vi "RT_AIChar_v3.vi"() -> ()   [LabVIEW 2020]
uses:
  <vilib>/NI/STM/SubVIs/MetaDataElement.ctl
  <vilib>/Platform/TimedLoop/XDataNode/timing_clust.ctl
  <vilib>/Platform/TimedLoop/XDataNode/nitl_modes.ctl
  <vilib>/Platform/TimedLoop/XDataNode/wakeup.ctl
  <vilib>/NI/STM/TCP/Write Meta Data (TCP Ref).vi
  <vilib>/NI/STM/TCP/Get Connection Reference (TCP).vi
  <vilib>/NI/STM/TCP/Write Meta Data (TCP Clst).vi
  <vilib>/FPGAPlugInAG/cRIO-9049/niLvFpga_Open_cRIO-9049.vi
  <vilib>/rvi/interface/common/dynamic/niFpgaDynamicAddResources.vi
  <vilib>/NI/STM/TCP/Write Message (TCP).vi
  <vilib>/Utility/error.llb/Error Cluster From Error Code.vi
  <vilib>/rvi/errors/niLvFpgaAdjustHostInterfaceError.vi
  <vilib>/FPGAPlugInAG/Dynamic/niLvFpga_Close_Dynamic.vi
  <vilib>/rvi/interface/nirviOpenFPGA/nirviOpenFPGA.xnode
  FPGA Bitfiles/levitationcode_FPGATarget_FPGAmainCtrlv4_ym4N2scWarI.lvbitx
  <vilib>/Platform/TimedLoop/XDataNode/XDataNode.xnode
  <vilib>/rvi/interface/nirviReadWriteControl/nirviReadWriteControl.xnode
  <vilib>/rvi/interface/nirviCloseFPGA/nirviCloseFPGA.xnode
  <vilib>/Platform/TimedLoop/XDataNode/XDNodeRunTimeDep.lvlib
  Components_global/Timing/Timing.lvlib
  <vilib>/NI/STM/NI STM.lvlib
  <vilib>/rvi/interface/Simulation/niFpgaSimulationCallBeginRW.vi
  NiFpgaLv.dll
panel:
  in  "Select channel":T1(ring)
  in  "Select HS or LS?":enum16{"HS (NI9222)", "LS (NI9220)"}(ring)
  out "RT Loop Rate":dbl format="%.3p"
  out "# of iterations\n[STM write]":i32
  out "# elements \nFIFO buffer":u32
  out "Finished \nlate counter?":dbl
  in  "stop":bool
  # "- Open PC_SensorChar vi and run that VI as well to start capturing data!"
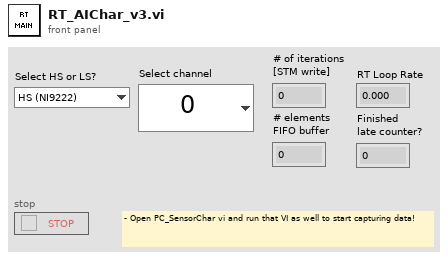
[diagram p1: front panel]
types:
  T1 = enum16{"0", "1", "2", "3", "4", "5", "6", "7", "8", "9", "10", "11", "12", "13", "14", "15"}
  T2 = typedef "NI STM.lvlib/MetaDataElement.ctl" = string
  T3 = typedef "NI STM.lvlib/TCP Connection Info.ctl" = cluster{"connection ID":refnum<k5>, "meta data":T2[]}
  T4 = typedef "XDNodeRunTimeDep.lvlib/timing_clust.ctl" = cluster{"Expected End [f-1]":u64, "Actual End [f-1]":u64, "Finished Late? [f-1]":bool, "Expected End [i-1]":u64, "Actual End [i-1]":u64, "Finished Late? [i-1]":bool, "Expected Start [i]":u64, "Actual Start [i]":u64, "Expected Start [f]":u64, "Actual Start [f]":u64, "Source Name":string, "Structure Name":string, "Period":i64, "Deadline":i64, "Offset":i64, "Start":i64, "Priority":i32, "Timeout":i32, "Mode":T5, "Wakeup Reason":T6, "Error":errorcluster, "Source Type":string, "Secondary Source Type":string, "Global End Time":u64, "Global Start Time":u64, "Frame Duration":u64, "Iteration Duration":u64, "Assigned CPU":i32, "I/O Scan Engine Mode":u32}
  T5 = typedef "XDNodeRunTimeDep.lvlib/nitl_modes.ctl" = enum32{"No Change", "Process missed periods, maintain original phase", "Discard missed periods, maintain original phase", "Process missed periods, ignore original phase", "Discard missed periods, ignore original phase"}
  T6 = typedef "XDNodeRunTimeDep.lvlib/wakeup.ctl" = enum32{"Normal", "Aborted", "Asynchronous wakeup", "Timing source error", "Timed loop error", "Timeout"}
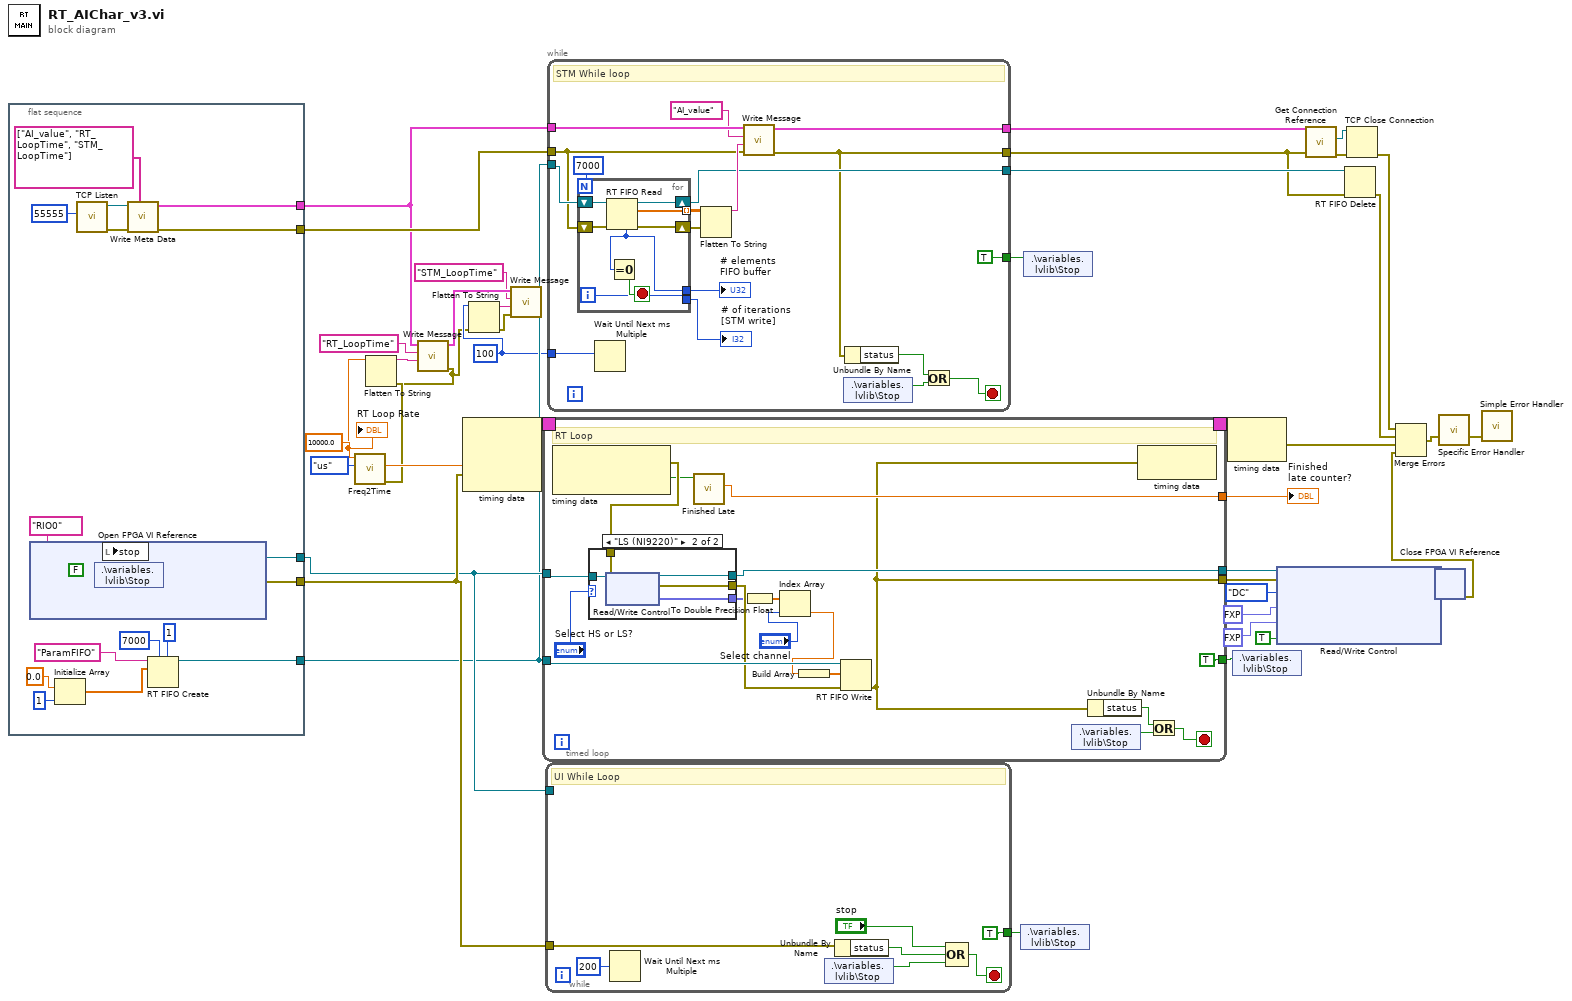
[diagram p0: block diagram]
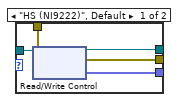
[diagram p2: hidden frame]
diagram:
  w11 = u32 100 ("millisecond multiple")
  n1 = flat-sequence {
    tunnel: [w59] -> w22
    tunnel: [w58] -> w21
    tunnel: [w53] -> w8
    tunnel: [w52] -> w37
    tunnel: [w51] -> w12
    frame #0 {
      w60 = FALSE ("Stop")
      n2 = xnode "Open FPGA VI Reference"("resource name"=tag "RIO0") -> ("FPGA VI Reference Out"=w58:refnum<k20>, "error out"=w61:errorcluster)  [unwired: 1 in]
      n3 = Initialize Array(0.0 ("element"), 1 ("dimension size")) -> (w46:dbl[])
      n4 = call <vilib>:"TCP Listen.vi"("port"=u16 55555) -> ("error out"=w56:errorcluster, "connection ID"=w55:refnum<k5>)  [unwired: 6 in, 3 out]
      n5 = shared-variable ".\\variables.lvlib\\Stop"(w60, error in=w61) -> (error out=w59:errorcluster)
      n6 = local write "stop"(w60) -> ()
      n7 = call-poly <vilib>:"Write Meta Data.vi"("meta data"=T2[] ["AI_value", "RT_LoopTime", "STM_LoopTime"], "error in"=w56, "connection ID"=w55) -> ("error out"=w52:errorcluster, "connection info out"=w53:T3)  [unwired: 7 in]
      n8 = RT FIFO Create(0:"ParamFIFO" ("name (unnamed)"), 1:w46, 4:u32 7000 ("size (10)"), 6:u32 1 ("elements in array (1)")) -> (8:w51:refnum<k33>)  [unwired: 4 in, 2 out]
    }
  }
  n9 = call "Freq2Time.vi"("Int. Time Unit"=enum16{"sec", "us", "ms"}."us", "Sample rate (Hz)"=10000.0 ("Period")) -> ("error out"=w26:errorcluster, "Int.  time [unit]"=w38:dbl, "New Sample rate (Hz)"=w28:dbl)  [unwired: 7 in]
  "RT Loop Rate" <- w28
  n10 = Flatten To String(anything=w28, error in (no error)=w26) -> (data string=w29:string, error out=w10:errorcluster)  [unwired: 2 in, 1 out]
  n11 = call-poly <vilib>:"Write Message.vi"("error in"=w10, "data"=w29, "name"="RT_LoopTime", "connection info in"=w8) -> ("connection info out"=w7:T3)  [unwired: 6 in, 1 out]
  n12 = node-c288(w38, w22) -> (w43:T4)  [unwired: 1 in]
  n13 = Flatten To String(anything=w11, error in (no error)=w10) -> (data string=w5:string, error out=w9:errorcluster)  [unwired: 2 in, 1 out]
  n14 = call-poly <vilib>:"Write Message.vi"("error in"=w9, "data"=w5, "name"="STM_LoopTime", "connection info in"=w7) -> ()  [unwired: 6 in, 2 out]
  n15 = timed-loop {
    tunnel: w21 -> [w79]
    timing: w43 -> [_]
    timing-out: [_] -> w42
    tunnel: [w76] -> w41
    tunnel: w12 -> [w75]
    tunnel: [TRUE ("Stop")] -> w14
    tunnel: [w67] -> w4
    tunnel: [w66] -> w3
    stop <- w73 stop-if-true
    # "RT Loop"
    n16 = node-c288() -> (w78:errorcluster, w77:bool)  [unwired: 1 in]
    n17 = case shown="\"LS (NI9220)\"" "Select HS or LS?" {
      tunnel: w79 -> [w84 w89]
      tunnel: w78 -> [w83 w88]
      tunnel: [w82 w87] -> w65
      tunnel: [w81 w86] -> w67
      tunnel: [w80 w85] -> w69
      frame "HS (NI9222)", Default {
        n18 = xnode "Read/Write Control"("FPGA VI Reference In"=w84, "error in"=w83) -> ("FPGA VI Reference Out"=w81:refnum<k20>, "error out"=w80:errorcluster, "AI_HS"=w82:fxp<+/-,25,5>[])
      }
      frame "LS (NI9220)" {
        n19 = xnode "Read/Write Control"("FPGA VI Reference In"=w89, "error in"=w88) -> ("FPGA VI Reference Out"=w86:refnum<k20>, "error out"=w85:errorcluster, "AI_LS"=w87:fxp<+/-,25,5>[])
      }
    }
    n20 = call "Finished Late.vi"("Finished \nLate?"=w77) -> ("# Finished\nLate counter"=w76:dbl)  [unwired: 8 in, 2 out]
    n21 = To Double Precision Float(number=w65) -> (double precision float=w64:dbl[])
    n22 = Index Array(array=w64, index="Select channel") -> (element=w63:dbl)
    n23 = Build Array(w63) -> (w62:dbl[])
    n24 = RT FIFO Write(0:w75, 1:w62, 3:w69) -> (11:w66:errorcluster)  [unwired: 2 in, 3 out]
    n25 = shared-variable ".\\variables.lvlib\\Stop"() -> (w72:bool)  [unwired: 1 in, 1 out]
    n26 = Unbundle By Name(w66) -> ("status"=w71:bool)
    n27 = node-c288(w66) -> ()  [unwired: 1 out]
    n28 = Or(x=w71, y=w72) -> (x .or. y?=w73:bool)
  }
  "Finished \nlate counter?" <- w41
  n29 = while {
    tunnel: w22 -> [w98]
    tunnel: w21 -> [_]
    tunnel: [TRUE ("Stop")] -> w13
    stop <- w99 stop-if-true
    # "UI While Loop"
    n30 = Wait Until Next ms Multiple(millisecond multiple=u32 200) -> ()  [unwired: 1 out]
    n31 = shared-variable ".\\variables.lvlib\\Stop"() -> (w100:bool)  [unwired: 1 in, 1 out]
    n32 = Unbundle By Name(w98) -> ("status"=w97:bool)
    n33 = Compound Arithmetic op=OR("stop", w97, w100) -> (w99:bool)
  }
  n34 = while {
    tunnel: w8 -> [w120]
    tunnel: w37 -> [w114]
    tunnel: [w118] -> w36
    tunnel: [w104] -> w32
    tunnel: w12 -> [w116]
    tunnel: [w113] -> w33
    tunnel: [TRUE ("Stop")] -> w15
    tunnel: w11 -> [w103]
    stop <- w106 stop-if-true
    # "STM While loop"
    n35 = for {
      N: 7000 -> [_]
      shift-right: [w125] -> w113
      shift-left: w116 -> [w128]
      shift-right: [w127] -> w115
      shift-left: w114 -> [w126]
      tunnel: [w124] -> w112
      tunnel: [w122] -> w111
      tunnel: [w121] -> w110 mode=indexing
      i -> [w122]
      stop <- w123 stop-if-true
      n36 = RT FIFO Read(0:w128, 3:w126) -> (7:w124:u32, 8:w125:refnum<k33>, 9:w121:dbl[], 11:w127:errorcluster)  [unwired: 2 in, 1 out]
      n37 = Equal To 0?(x=w124) -> (x = 0?=w123:bool)
    }
    "# elements \nFIFO buffer" <- w112
    "# of iterations\n[STM write]" <- w111
    n38 = Wait Until Next ms Multiple(millisecond multiple=w103) -> ()  [unwired: 1 out]
    n39 = Flatten To String(anything=w110, error in (no error)=w115) -> (data string=w117:string)  [unwired: 2 in, 2 out]
    n40 = call-poly <vilib>:"Write Message.vi"("error in"=w114, "data"=w117, "name"="AI_value", "connection info in"=w120) -> ("error out"=w104:errorcluster, "connection info out"=w118:T3)  [unwired: 6 in]
    n41 = shared-variable ".\\variables.lvlib\\Stop"() -> (w107:bool)  [unwired: 1 in, 1 out]
    n42 = Unbundle By Name(w104) -> ("status"=w105:bool)
    n43 = Or(x=w105, y=w107) -> (x .or. y?=w106:bool)
  }
  n44 = shared-variable ".\\variables.lvlib\\Stop"(w13) -> ()  [unwired: 1 in, 1 out]
  n45 = shared-variable ".\\variables.lvlib\\Stop"(w15) -> ()  [unwired: 1 in, 1 out]
  n46 = node-c288(w42) -> (w27:errorcluster)
  n47 = shared-variable ".\\variables.lvlib\\Stop"(w14) -> ()  [unwired: 1 in, 1 out]
  n48 = xnode "Read/Write Control"("FPGA VI Reference In"=w4, "error in"=w3, "PR Excitation mode"=enum8{"DC", "Sine", "Square", "WhiteNoise"}."DC", "PR Amplitude [V]"=fxp<+/-,25,5> 0.0 ("Amplitude [V]"), "PR Frequency [periods/tick]"=fxp<+,32,0> 0.0 ("Frequency [periods/tick]"), "Enable  Pos. Ref. Gen?"=TRUE) -> ("FPGA VI Reference Out"=w19:refnum<k20>, "error out"=w18:errorcluster)
  n49 = call-poly <vilib>:"Get Connection Reference.vi"("error in"=w32, "connection info in"=w36) -> ("error out"=w35:errorcluster, "connection ID out"=w34:refnum<k5>)  [unwired: 7 in, 1 out]
  n50 = RT FIFO Delete(0:w33, 3:w32) -> (11:w31:errorcluster)  [unwired: 1 in]
  n51 = TCP Close Connection(connection ID=w34, error in (no error)=w35) -> (error out=w23:errorcluster)  [unwired: 1 in, 1 out]
  n52 = xnode "Close FPGA VI Reference"("FPGA VI Reference In"=w19, "error in"=w18) -> ("error out"=w20:errorcluster)
  n53 = Merge Errors(w23, w31, w27, w20) -> (w25:errorcluster)
  n54 = call "Specific Error Handler"("Error to Check"=w25) -> ("error out"=w24:errorcluster)  [unwired: 11 in, 3 out]
  n55 = call <vilib>:"Simple Error Handler.vi"("error in (no error)"=w24) -> ()  [unwired: 4 in, 5 out]
